vi "Initialize Instrument.vi"(8 "error in (no error)":errorcluster, 10 "Instr Resource Str":string, 11 "NI Digitizer.lvclass in":refnum<class "NI Digitizer.lvclass">) -> (0 "error out":errorcluster, 3 "NI Digitizer.lvclass out":refnum<class "NI Digitizer.lvclass">)   [LabVIEW 2010, in "NI Digitizer.lvclass"]
uses:
  NI Digitizer.lvclass
  NI Digitizer.lvclass/NI Digitizer.ctl
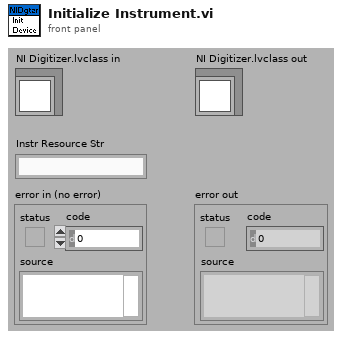
[diagram p1: front panel]
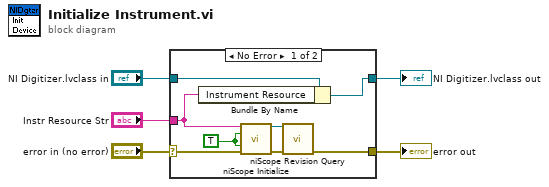
[diagram p0: block diagram]
diagram:
  n1 = case shown="No Error" "error in (no error)" {
    selector: "error in (no error)" -> [w9 w14]
    tunnel: [w6 w15] -> w4
    tunnel: [w11 w14] -> w5
    tunnel: "NI Digitizer.lvclass in" -> [w8 w15]
    tunnel: "Instr Resource Str" -> [w7 _]
    frame No Error {
      w13 = TRUE ("ID Query? (T: Yes)")
      n2 = Bundle By Name(cluster=w8, "Instrument Resource"=w7) -> (w6:refnum<class "NI Digitizer.lvclass">)
      n3 = call <instrlib>:"niScope Initialize.vi"("resource name"=w7, "id query"=w13, "reset device"=w13, "error in"=w9) -> ("instrument handle"=w10:refnum<k15>, "error out"=w12:errorcluster)  [unwired: 10 out]
      n4 = call <instrlib>:"niScope Revision Query.vi"("instrument handle"=w10, "error in"=w12) -> ("error out"=w11:errorcluster)  [unwired: 13 out]
    }
    frame Error {
    }
  }
  "error out" <- w5
  "NI Digitizer.lvclass out" <- w4
